vi "rvc Plot 2D Transform (scalar).vi"(8 "Error In":errorcluster, 11 "T":dbl[][](array[numeric])=[[-0.4161468365471424, 0.9092974268256817, 3.0], [-0.9092974268256817, -0.4161468365471424, 1.0], [0.0, 0.0, 1.0]]) -> (0 "Error Out":errorcluster, 3 "XY Graph 2":cluster{dbl[], dbl[]}(graph))   [LabVIEW 2017]
doc: "Given a 3x3 homogenous transformation (T) this function outputs a cluster of the plot components (TrPlot) needed to represent the transformation on an XY Graph."
uses:
  <vilib>/Analysis/coordinate.llb/2D Cartesian Coordinate Rotation (Scalar).vi
  <vilib>/Analysis/NI_AALPro.lvlib
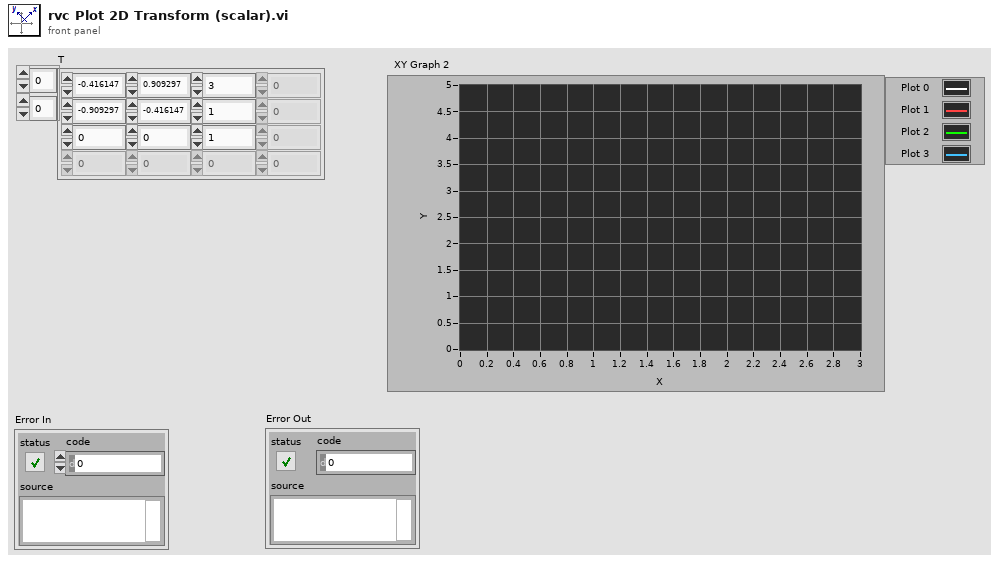
[diagram p1: front panel]
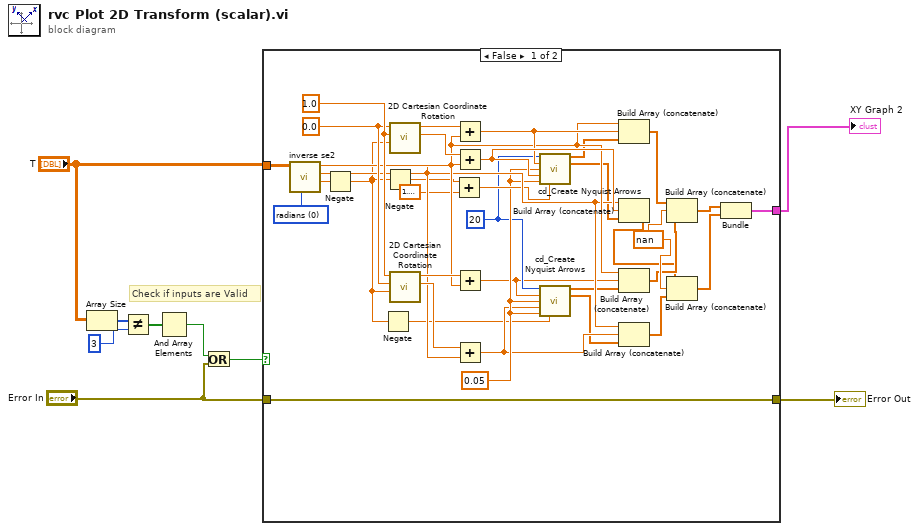
[diagram p0: block diagram]
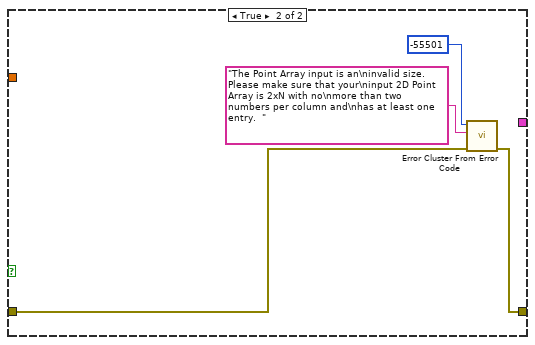
[diagram p2: hidden frame]
diagram:
  # "Check if inputs are Valid"
  n1 = Array Size(array="T") -> (size(s)=w8:i32[])
  n2 = Not Equal?(x=w8, y=3) -> (x != y?=w2:bool[])
  n3 = And Array Elements(Boolean array=w2) -> (logical AND=w1:bool)
  n4 = Or(x=w1, y="Error In") -> (x .or. y?=w7:bool)
  n5 = case shown="False" w7 {
    tunnel: "T" -> [w41 _]
    tunnel: [w42 _] -> w5
    tunnel: "Error In" -> [w43 w46]
    tunnel: [w43 w45] -> w6
    frame False {
      w11 = u16 0 items=["radians", "degree"] ("angle unit")
      w15 = nan
      w32 = 0.0 ("element")
      w33 = 1.0 ("element")
      w25 = 0.05 ("dx")
      w24 = 20 ("number of arrows")
      n6 = call "inverse se2.vi"("angle unit"=w11, "T"=w41) -> ("theta"=w22:dbl, "y"=w29:dbl, "x"=w30:dbl)  [unwired: 6 in, 1 out]
      n7 = Negate(x=w22) -> (-x=w10:dbl)
      n8 = Negate(x=w10) -> (-x=w16:dbl)
      n9 = Negate(x=w10) -> (-x=w17:dbl)
      n10 = call-poly <vilib>:"2D Cartesian Coordinate Rotation.vi"("theta"=w10, "y"=w33, "x"=w32) -> ("y out"=w34:dbl, "x out"=w38:dbl)  [unwired: 6 in, 1 out]
      n11 = call-poly <vilib>:"2D Cartesian Coordinate Rotation.vi"("theta"=w10, "y"=w32, "x"=w33) -> ("y out"=w39:dbl, "x out"=w40:dbl)  [unwired: 6 in, 1 out]
      n12 = Add(x=w17, y=1.5707963267948966) -> (x+y=w28:dbl)
      n13 = Add(x=w38, y=w30) -> (x+y=w31:dbl)
      n14 = Add(x=w34, y=w29) -> (x+y=w35:dbl)
      n15 = Add(x=w40, y=w30) -> (x+y=w23:dbl)
      n16 = Add(x=w39, y=w29) -> (x+y=w21:dbl)
      n17 = call <vilib>:"cd_Create Nyquist Arrows.vi"("number of arrows"=w24, "xo"=w31, "dx"=w25, "yo"=w35, "dy"=w25, "theta"=w28) -> ("array of x"=w27:dbl[], "array of y"=w26:dbl[])  [unwired: 8 in]
      n18 = call <vilib>:"cd_Create Nyquist Arrows.vi"("number of arrows"=w24, "xo"=w23, "dx"=w25, "yo"=w21, "dy"=w25, "theta"=w16) -> ("array of x"=w19:dbl[], "array of y"=w18:dbl[])  [unwired: 8 in]
      n19 = Build Array (concatenate)(w30, w31, w27) -> (w44:dbl[])
      n20 = Build Array (concatenate)(w29, w35, w26) -> (w13:dbl[])
      n21 = Build Array (concatenate)(w30, w23, w19) -> (w14:dbl[])
      n22 = Build Array (concatenate)(w29, w21, w18) -> (w12:dbl[])
      n23 = Build Array (concatenate)(w44, w15, w14) -> (w37:dbl[])
      n24 = Build Array (concatenate)(w13, w15, w12) -> (w36:dbl[])
      n25 = Bundle(w37, w36) -> (w42:cluster{dbl[], dbl[]})  [unwired: 1 in]
    }
    frame True {
      n26 = call <vilib>:"Error Cluster From Error Code.vi"("error in (no error)"=w46, "error message (\"\")"="The Point Array input is an\ninvalid size. Please make sure that your\ninput 2D Point Array is 2xN with no\nmore than two numbers per column and\nhas at least one entry.  " ("error message (\"\")"), "error code (0)"=-55501) -> ("error out"=w45:errorcluster)  [unwired: 6 in]
    }
  }
  "Error Out" <- w6
  "XY Graph 2" <- w5
